vi "VI Clipboard Copy.vi"(8 "error in (no error)":errorcluster, 10 "Selection List Only? (F=All)":bool, 11 "VI Refnum in":refnum<vi>) -> (0 "error out":errorcluster, 3 "dup VI Refnum":refnum<vi>)   [LabVIEW 2022 SP3, in "VI-Snippet.lvlib"]
doc: "Copies the <b>VI Refnum in</b> block diagram content to the clipboard. If <b>Selected GObjects Only?</b> is True, this only copies the currently selected GObjects on the block diagram. Otherwise, all diagram content is copied."
uses:
  VI-Snippet.lvlib
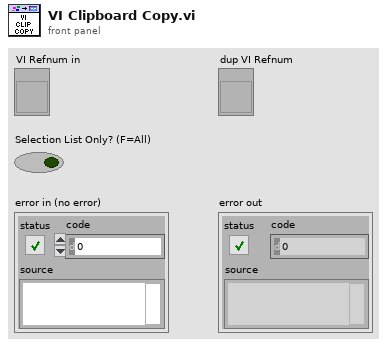
[diagram p1: front panel]
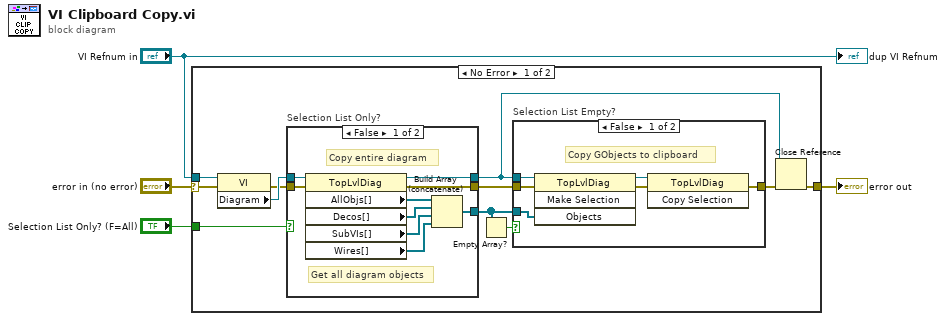
[diagram p0: block diagram]
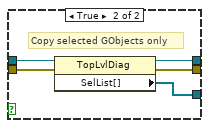
[diagram p2: hidden frame]
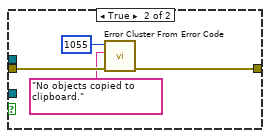
[diagram p3: hidden frame]
diagram:
  n1 = case shown="No Error" "error in (no error)" {
    selector: "error in (no error)" -> [w11 w40]
    tunnel: "VI Refnum in" -> [w10 _]
    tunnel: [w9 w40] -> w3
    tunnel: "Selection List Only? (F=All)" -> [w8 _]
    frame No Error {
      n2 = property class="VI"(reference=w10, error in=w11) -> (error out=w13:errorcluster, "Diagram"=w15:refnum<vi>)  [unwired: 1 out]
      n3 = case "Selection List Only?" shown="False" w8 {
        tunnel: w15 -> [w24 w27]
        tunnel: [w23 w25] -> w14
        tunnel: w13 -> [w22 w29]
        tunnel: [w21 w28] -> w12
        tunnel: [w16 w26] -> w6
        frame False {
          # "Copy entire diagram"
          # "Get all diagram objects"
          n4 = property class="TopLvlDiag"(reference=w24, error in=w22) -> (reference out=w23:refnum<vi>, error out=w21:errorcluster, "AllObjs[]"=w20:refnum<vi>[], "Decos[]"=w19:refnum<vi>[], "SubVIs[]"=w18:refnum<vi>[], "Wires[]"=w17:refnum<vi>[])
          n5 = Build Array (concatenate)(w20, w19, w18, w17) -> (w16:refnum<vi>[])
        }
        frame True {
          # "Copy selected GObjects only"
          n6 = property class="TopLvlDiag"(reference=w27, error in=w29) -> (reference out=w25:refnum<vi>, error out=w28:errorcluster, "SelList[]"=w26:refnum<vi>[])
        }
      }
      n7 = Empty Array?(array=w6) -> (empty?=w7:bool)
      n8 = case "Selection List Empty?" shown="False" w7 {
        tunnel: w14 -> [w35 _]
        tunnel: w12 -> [w34 w39]
        tunnel: [w30 w38] -> w5
        tunnel: w6 -> [w31 _]
        frame False {
          # "Copy GObjects to clipboard"
          n9 = invoke class="TopLvlDiag" method="Make Selection"(reference=w35, error in=w34, "Objects"=w31) -> (reference out=w32:refnum<vi>, error out=w33:errorcluster)  [unwired: 1 in, 2 out]
          n10 = invoke class="TopLvlDiag" method="Copy Selection"(reference=w32, error in=w33) -> (error out=w30:errorcluster)  [unwired: 1 in, 2 out]
        }
        frame True {
          n11 = call <vilib>:"Error Cluster From Error Code.vi"("error in (no error)"=w39, "error message (\"\")"="No objects copied to clipboard.", "error code (0)"=1055) -> ("error out"=w38:errorcluster)  [unwired: 6 in]
        }
      }
      n12 = Close Reference(reference=w14, error in (no error)=w5) -> (error out=w9:errorcluster)
    }
    frame Error {
    }
  }
  "error out" <- w3
  "dup VI Refnum" <- "VI Refnum in"
